vi "Freeze Value.vi"(1 "Freeze Value":bool, 2 "In Value":dbl) -> (0 "Value Out":dbl)   [LabVIEW 2012]
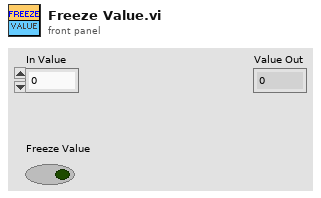
[diagram p1: front panel]
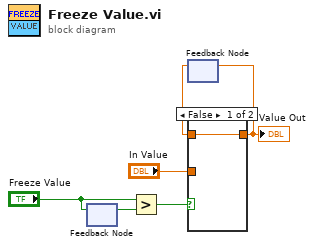
[diagram p0: block diagram]
diagram:
  n1 = feedback #1() -> (w6:bool)  [unwired: 1 in]
  n2 = feedback-in #1("Freeze Value") -> ()
  n3 = Greater?(x="Freeze Value", y=w6) -> (0:w4:bool)
  n4 = feedback #2() -> (w3:dbl)  [unwired: 1 in]
  n5 = case shown="False" w4 {
    tunnel: "In Value" -> [_ w8]
    tunnel: w3 -> [w7 _]
    tunnel: [w7 w8] -> w2
    frame False {
    }
    frame True {
    }
  }
  "Value Out" <- w2
  n6 = feedback-in #2(w2) -> ()
